vi "SubscriberCallbackInternal.vi"(4 "Message":refnum<user-event>, 5 "Event Data":cluster{"sender":refnum<k24>, "e":refnum<k24>}, 6 "Control Ref":refnum<k24>, 7 "Event Common Data":T1) -> ()   [LabVIEW 2017]
uses:
  C:/Program Files (x86)/National Instruments/LabVIEW 2017/vi.lib/addons/InsightCM/Binaries/LabviewMessageAdapter.dll
  Binaries/LabviewMessageAdapter.dll
  <vilib>/addons/InsightCM/MessageBus/Base/controls/MessageWrapper.ctl
  <vilib>/addons/InsightCM/MessageBus/Base/controls/Message.ctl
  <vilib>/addons/InsightCM/MessageBus/Base/controls/MessageHeader.ctl
  <vilib>/addons/InsightCM/MessageBus/Base/controls/KeyValuePair.ctl
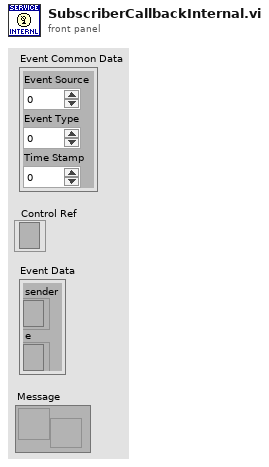
[diagram p1: front panel]
types:
  T1 = cluster{"Event Source":i32, "Event Type":u32, "Time Stamp":u32}
  T2 = typedef "MessageWrapper.ctl" = cluster{"Message":T3}
  T3 = typedef "Message.ctl" = cluster{"Header":T4, "Body":u8[]}
  T4 = typedef "MessageHeader.ctl" = cluster{"MessageName":string, "Timestamp":i64, "CorrelationId":string, "ContentType":string, "RoutingKey":string, "Properties":T5[]}
  T5 = typedef "KeyValuePair.ctl" = cluster{"Key":string, "Value":string}
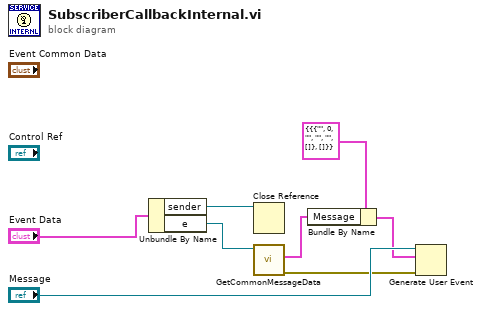
[diagram p0: block diagram]
diagram:
  n1 = Unbundle By Name("Event Data") -> ("sender"=w8:refnum<k24>, "e"=w7:refnum<k24>)
  n2 = Close Reference(reference=w8) -> ()  [unwired: 1 in, 1 out]
  n3 = call <vilib>:"GetCommonMessageData.vi"("MessageArgs"=w7) -> ("error out"=w4:errorcluster, "Message"=w2:T3)  [unwired: 8 in, 1 out]
  n4 = Bundle By Name(cluster=T2 {"Message"={"Header"={"MessageName"="", "Timestamp"=0, "CorrelationId"="", "ContentType"="", "RoutingKey"="", "Properties"=[]}, "Body"=[]}} ("Message"), "Message"=w2) -> (w1:T2)
  n5 = Generate User Event(user event="Message", event data cluster=w1, error in=w4) -> ()  [unwired: 1 in, 2 out]
